vi "Write NET_StreamContent.vi"(8 "error in (no error)":errorcluster, 10 "NET_StreamContent":refnum<k24>, 11 "HttpContent_Stream in":refnum<class "HttpContent_Stream.lvclass">) -> (0 "error out":errorcluster, 3 "HttpContent_Stream out":refnum<class "HttpContent_Stream.lvclass">)   [LabVIEW 2018, in "HttpClient_NET.lvlib" / "HttpContent_Stream.lvclass"]
doc: "<b> </b> <b> </b>\nHttpClient_NET\nJustin Young - Viviota\nCopyright (c) 2021\nLicense: BSD"
uses:
  HttpContent_Stream.lvclass
  C:/Viviota/Projects/R&D/__OpenSource/VIV_HTTP_REST_NET/HttpContent/HttpContent.lvclass
  System.Net.Http
  HttpContent/HttpContent.lvclass/HttpContent.ctl
  HttpContent/HttpContent.lvclass
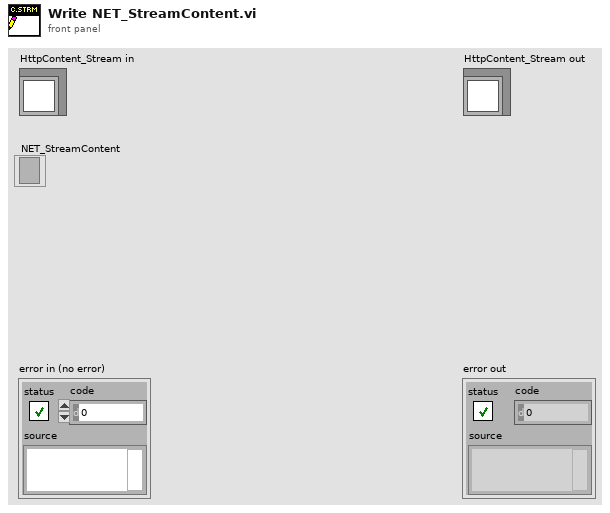
[diagram p1: front panel]
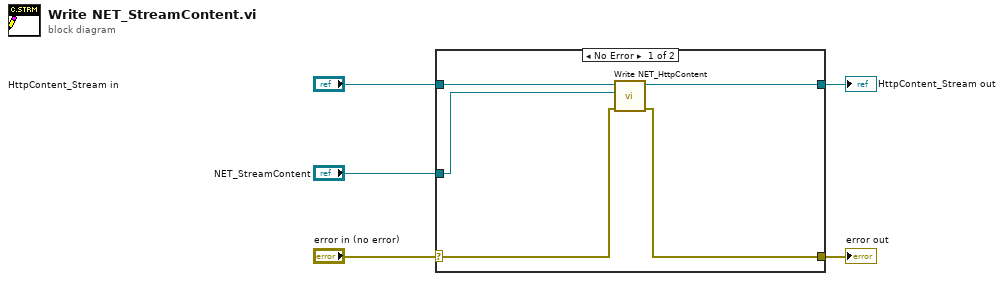
[diagram p0: block diagram]
diagram:
  n1 = case shown="No Error" "error in (no error)" {
    selector: "error in (no error)" -> [w7 w11]
    tunnel: [w6 w11] -> w4
    tunnel: [w9 w12] -> w2
    tunnel: "HttpContent_Stream in" -> [w10 w12]
    tunnel: "NET_StreamContent" -> [w8 _]
    frame No Error {
      n2 = call "Write NET_HttpContent.vi"("error in (no error)"=w7, "NET_HttpContent"=w8, "HttpContent in"=w10) -> ("error out"=w6:errorcluster, "HttpContent out"=w9:refnum<class "HttpContent_Stream.lvclass">)  [unwired: 7 in]
    }
    frame Error {
    }
  }
  "error out" <- w4
  "HttpContent_Stream out" <- w2
